vi "Close.vi"(8 "error in (no error)":errorcluster, 11 "ArrayController in":refnum<class "ArrayController.lvclass">) -> (0 "error out":errorcluster, 3 "ArrayController out":refnum<class "ArrayController.lvclass">)   [LabVIEW 2018, in "ArrayController.lvclass"]
uses:
  ArrayController.lvclass
  ArrayController.lvclass/ArrayController.ctl
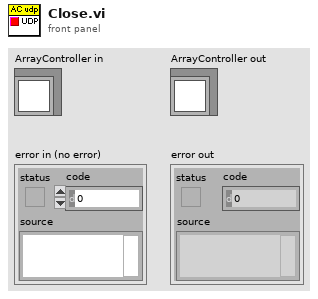
[diagram p1: front panel]
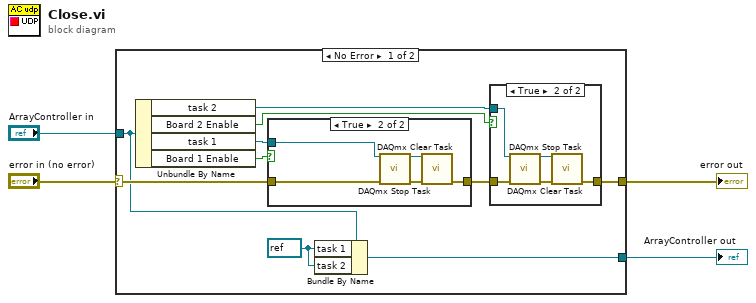
[diagram p0: block diagram]
diagram:
  n1 = case shown="No Error" "error in (no error)" {
    selector: "error in (no error)" -> [w12 w28]
    tunnel: [w8 w28] -> w3
    tunnel: [w6 w27] -> w1
    tunnel: "ArrayController in" -> [w7 w27]
    frame No Error {
      w5 = refnum<k21> refnum ("task 1")
      n2 = Unbundle By Name(w7) -> ("task 2"=w9:refnum<k21>, "Board 2 Enable"=w10:bool, "task 1"=w14:refnum<k21>, "Board 1 Enable"=w13:bool)
      n3 = case shown="True" w13 {
        tunnel: w14 -> [_ w25]
        tunnel: w12 -> [w21 w24]
        tunnel: [w21 w23] -> w11
        frame False {
        }
        frame True {
          n4 = call <vilib>:"DAQmx Stop Task.vi"("task/channels in"=w25, "error in"=w24) -> ("task out"=w22:refnum<k21>, "error out"=w26:errorcluster)  [unwired: 12 in]
          n5 = call <vilib>:"DAQmx Clear Task.vi"("task in"=w22, "error in"=w26) -> ("error out"=w23:errorcluster)  [unwired: 13 in]
        }
      }
      n6 = Bundle By Name(cluster=w7, "task 1"=w5, "task 2"=w5) -> (w6:refnum<class "ArrayController.lvclass">)
      n7 = case shown="True" w10 {
        tunnel: w9 -> [_ w19]
        tunnel: w11 -> [w15 w18]
        tunnel: [w15 w17] -> w8
        frame False {
        }
        frame True {
          n8 = call <vilib>:"DAQmx Stop Task.vi"("task/channels in"=w19, "error in"=w18) -> ("task out"=w16:refnum<k21>, "error out"=w20:errorcluster)  [unwired: 12 in]
          n9 = call <vilib>:"DAQmx Clear Task.vi"("task in"=w16, "error in"=w20) -> ("error out"=w17:errorcluster)  [unwired: 13 in]
        }
      }
    }
    frame Error {
    }
  }
  "error out" <- w3
  "ArrayController out" <- w1
